vi "SeCrTs-DI Data.vi"(7 "Enum":enum16{"Write", "Read"}(ring), 11 "In_DI data":digitalwaveform[](array[waveform])) -> (3 "Out_DI data":digitalwaveform[](array[waveform]))   [LabVIEW 2022 SP3]
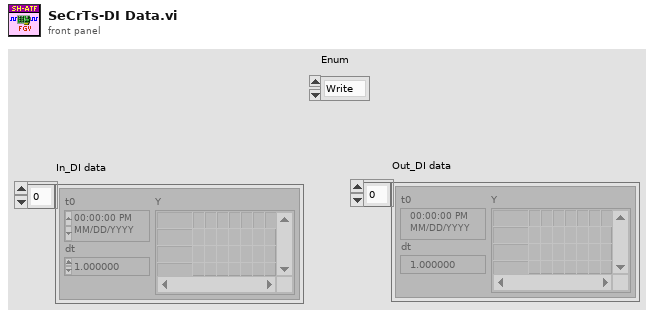
[diagram p1: front panel]
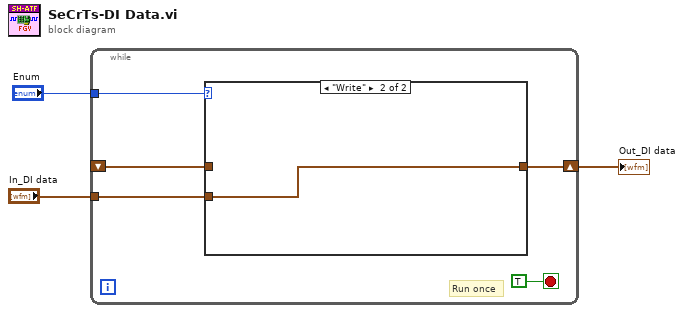
[diagram p0: block diagram]
diagram:
  n1 = while {
    tunnel: "Enum" -> [w7]
    tunnel: "In_DI data" -> [w6]
    shift-right: [w5] -> w1
    shift-left: _ -> [w4]
    stop <- TRUE stop-if-true
    # "Run once"
    n2 = case shown="\"Write\"" w7 {
      tunnel: w6 -> [_ w10]
      tunnel: [w9 w10] -> w5
      tunnel: w4 -> [w9 _]
      frame "Read" {
      }
      frame "Write" {
      }
    }
  }
  "Out_DI data" <- w1
